vi "QMASSdll.vi"(8 "error in (no error)":errorcluster, 11 "Inputs":cluster{"qmol":dbl, "x":dbl[], "y":dbl[]}) -> (0 "error out":errorcluster, 3 "Outputs":T1)   [LabVIEW 2016]
doc: "subroutine QMASSdll(qmol, x, y, qkg, xlkg, xvkg, wliq, wvap, ierr, herr, herr_length)\n\nConverts quality and composition on a mole basis to a mass basis.\n\nINPUTS:\nqmol -- molar quality [moles vapor/total moles]\n qmol = 0 indicates saturated liquid\n qmol = 1 indicates saturated vapor\n 0 < qmol < 1 indicates a two-phase state\n qmol < 0 or qmol > 1 are not allowed and will result in warning\nx -- composition of liquid phase [array of mol frac]\ny --composition of vapor phase [array of mol frac]\n\nOUTPUTS:\nqkg -- quality on mass basis [mass of vapor/total mass]\nxlkg -- mass composition of liquid phase [array of mass frac]\nxvkg -- mass composition of vapor phase [array of mass frac]\nwliq -- molecular weight of liquid phase [g/mol]\nwvap -- molecular weight of vapor phase [g/mol]\nierr -- Error flag: 0 - All inputs within limits -19 - Input q < 0 or > 1\nherr -- Error string (character*255)\nherr_length -- length of variable herr (default: 255)"
uses:
  REFPROP.DLL
panel:
  # "REFPROP-QMASSdll.vi"
  # "void  QMASSdll(double *qmol, double *x, double *y, double *qkg, double *xlkg, double *xvkg, double *wliq, double *wvap, int32_t *ierr, CStr herr, int32_t herr_length)"
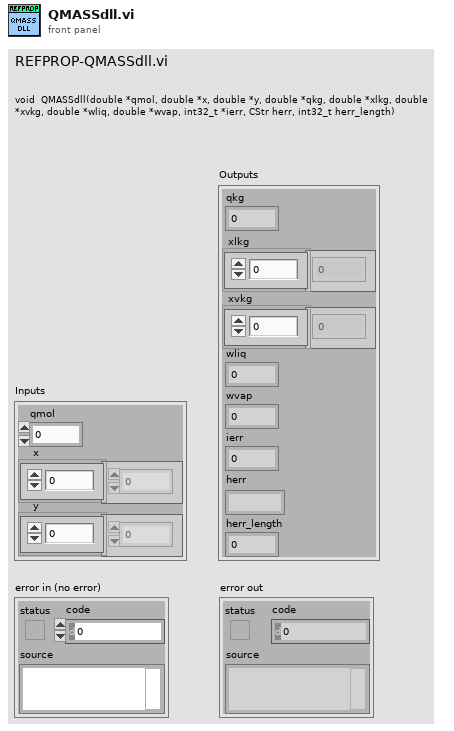
[diagram p1: front panel]
types:
  T1 = cluster{"qkg":dbl, "xlkg":dbl[], "xvkg":dbl[], "wliq":dbl, "wvap":dbl, "ierr":i32, "herr":string, "herr_length":i32}
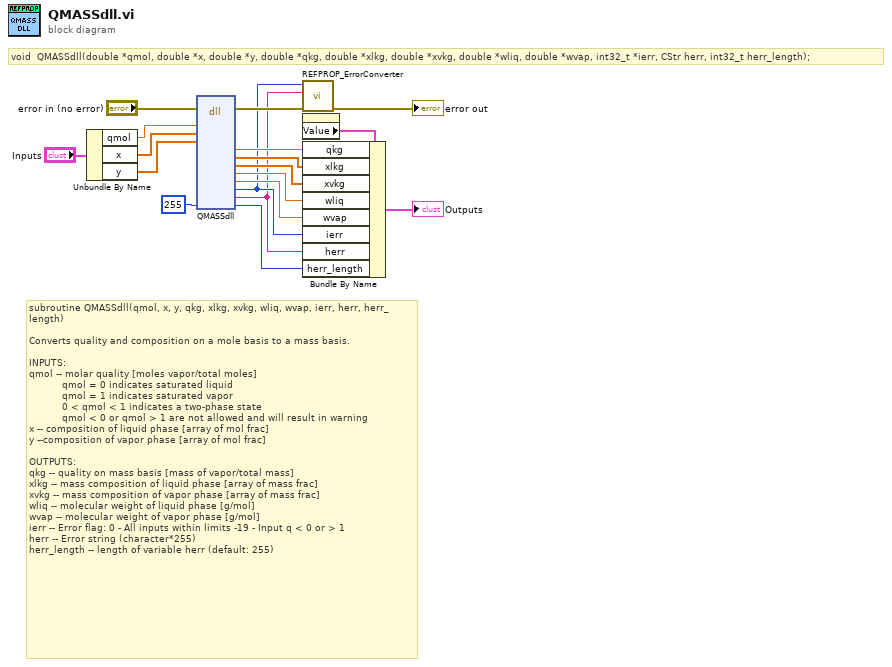
[diagram p0: block diagram]
diagram:
  # "void  QMASSdll(double *qmol, double *x, double *y, double *qkg, double *xlkg, double *xvkg, double *wliq, double *wvap, int32_t *ierr, CStr herr, int32_t herr_length);"
  # "subroutine QMASSdll(qmol, x, y, qkg, xlkg, xvkg, wliq, wvap, ierr, herr, herr_length)\n\nConverts quality and composition on a mole basis to a mass basis.\n\nINPUTS:\nqmol -- molar quality [moles vapor/total moles]\n           qmol = 0 indicates saturated liquid\n           qmol = 1 indicates saturated vapor\n           0 < qmol < 1 indicates a two-phase state\n           qmol < 0 or qmol > 1 are not allowed and will result in warning\nx -- composition of liquid phase [array of mol frac]\ny --composition of vapor phase [array of mol frac]\n\nOUTPUTS:\nqkg -- quality on mass basis [mass of vapor/total mass]\nxlkg -- mass composition of liquid phase [array of mass frac]\nxvkg -- mass composition of vapor phase [array of mass frac]\nwliq -- molecular weight of liquid phase [g/mol]\nwvap -- molecular weight of vapor phase [g/mol]\nierr -- Error flag: 0 - All inputs within limits -19 - Input q < 0 or > 1\nherr -- Error string (character*255)\nherr_length -- length of variable herr (default: 255)"
  n1 = Unbundle By Name("Inputs") -> ("qmol"=w13:dbl, "x"=w12:dbl[], "y"=w11:dbl[])
  n2 = dll-call lib="S:/009 - Testing/02 - Performance Testing/REFPROP/REFPROP.*" fn="QMASSdll"(error in="error in (no error)", "qmol"=w13, "x"=w12, "y"=w11, "herr_length"=255 ("ln")) -> (error out=w17:errorcluster, "qkg"=w4:dbl, "xlkg"=w5:dbl[], "xvkg"=w6:dbl[], "wliq"=w7:dbl, "wvap"=w8:dbl, "ierr"=w2:i32, "herr"=w1:string, "herr_length"=w9:i32)  [unwired: 13 in, 1 out]
  n3 = call "REFPROP_ErrorConverter.vi"("error in (no error)"=w17, "Error Message"=w1, "Error Code"=w2) -> ("error out"=→"error out":errorcluster)  [unwired: 8 in]
  n4 = property on="Outputs" class="Clust (strict)"() -> ("Value"=w10:T1)  [unwired: 2 in, 2 out]
  n5 = Bundle By Name(cluster=w10, "qkg"=w4, "xlkg"=w5, "xvkg"=w6, "wliq"=w7, "wvap"=w8, "ierr"=w2, "herr"=w1, "herr_length"=w9) -> (→"Outputs":T1)
